vi "SaveArrayToTxt.vi"(1 "Input array":dbl[][](array[numeric]), 3 "Filename":string="Trial_sequence", 4 "File path":path=path "D:/Data/trackingresults") -> (0 "Boolean":bool=TRUE)   [LabVIEW 2013]
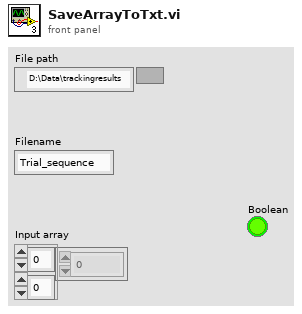
[diagram p1: front panel]
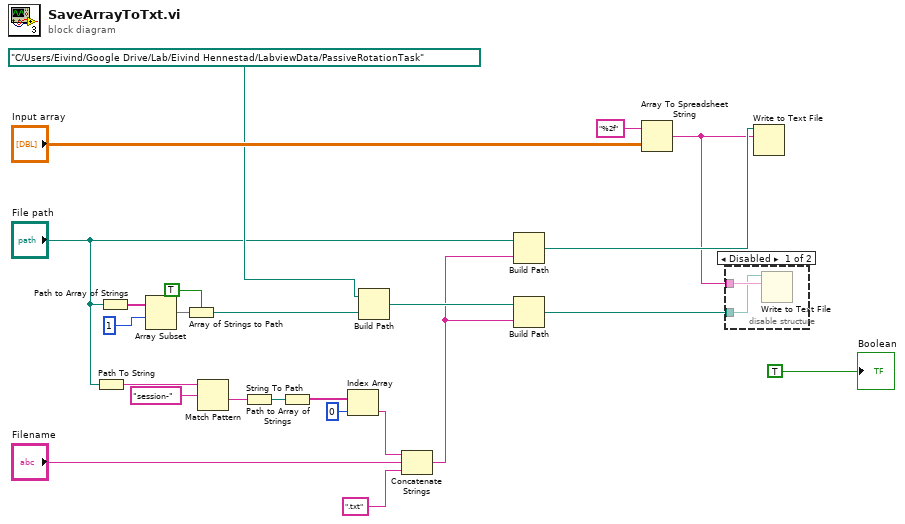
[diagram p0: block diagram]
diagram:
  n1 = Path To String(path="File path") -> (string=w1:string)
  n2 = Path to Array of Strings(0:"File path") -> (2:w12:string[])  [unwired: 1 out]
  n3 = Array Subset(array=w12, index=1) -> (w10:string[])  [unwired: 1 in]
  n4 = Array of Strings to Path(0:w10, 1:TRUE ("relative")) -> (2:w9:path)
  n5 = Match Pattern(string=w1, regular expression="session-") -> (after substring=w7:string)  [unwired: 1 in, 3 out]
  n6 = String To Path(string=w7) -> (path=w6:path)
  n7 = Path to Array of Strings(0:w6) -> (2:w5:string[])  [unwired: 1 out]
  n8 = Index Array(array=w5, index=0) -> (element=w3:string)
  n9 = Build Path(base path=path "C:/Users/Eivind/Google Drive/Lab/Eivind Hennestad/LabviewData/PassiveRotationTask", name or relative path=w9) -> (appended path=w18:path)
  n10 = Concatenate Strings(w3, "Filename", ".txt" ("string")) -> (w17:string)
  n11 = Build Path(base path="File path", name or relative path=w17) -> (appended path=w23:path)
  n12 = Build Path(base path=w18, name or relative path=w17) -> (appended path=w15:path)
  n13 = Array To Spreadsheet String(array="Input array", 3:"%2f" ("format string")) -> (spreadsheet string=w16:string)  [unwired: 1 in]
  n14 = disable-structure shown="Disabled" {
    disable-tunnel: w16 -> [w26 _]
    disable-tunnel: w15 -> [w25 _]
    frame Disabled {
      n15 = Write to Text File(file (use dialog)=w25, text=w26) -> ()  [unwired: 2 in, 3 out]
    }
    frame Enabled {
    }
  }
  n16 = Write to Text File(file (use dialog)=w23, text=w16) -> ()  [unwired: 2 in, 3 out]
  "Boolean" <- TRUE
